vi "Calculate schedules time.vi"(8 "error in (no error)":errorcluster) -> (0 "error out":errorcluster)   [LabVIEW 2020]
uses:
  <vilib>/Utility/miscctls.llb/LVDateTimeRec.ctl
  Global variable.vi
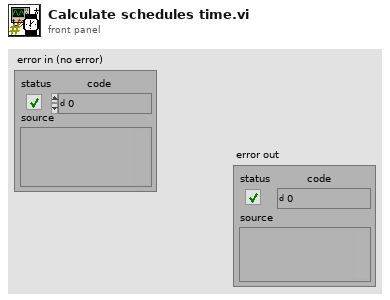
[diagram p1: front panel]
types:
  T1 = typedef "LVDateTimeRec.ctl" = cluster{"fractional second":dbl, "second":i32, "minute":i32, "hour":i32, "day of month":i32, "month":i32, "year":i32, "day of week":i32, "day of year":i32, "DST":i32}
  T2 = typedef "Schedule.ctl" = cluster{"Start time":timestamp, "Repeat":T3, "Action":T4}
  T3 = typedef "Repeat.ctl" = enum16{"None", "Every hour", "Every day", "Every week", "Every month"}
  T4 = typedef "Action.ctl" = u16
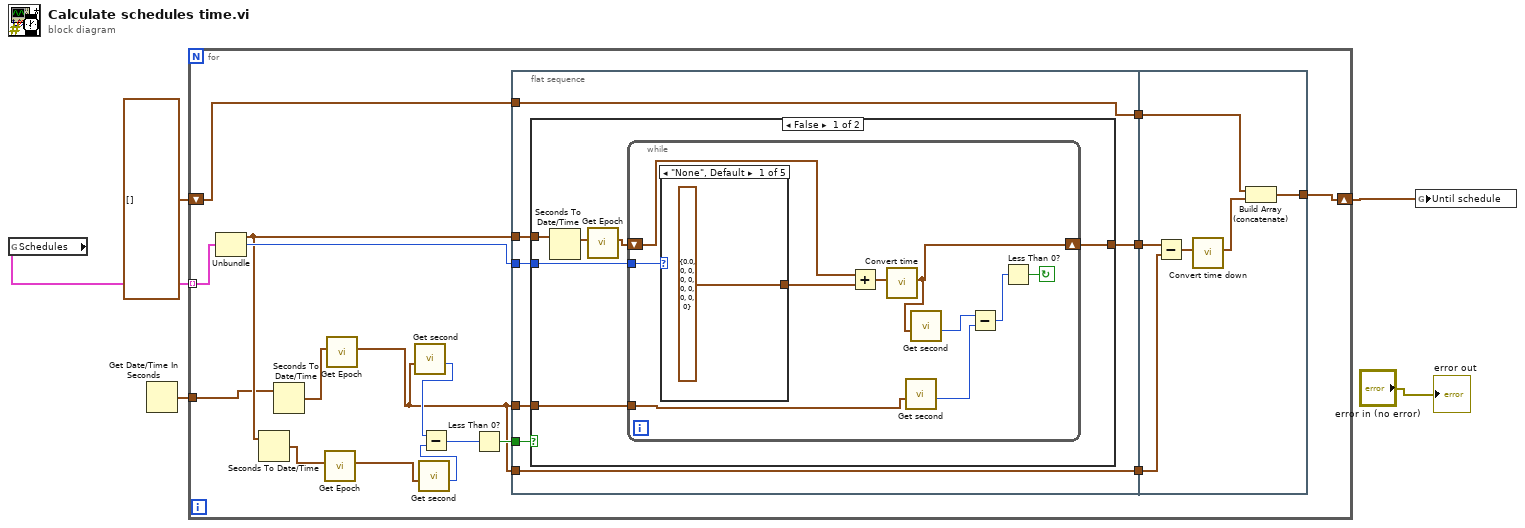
[diagram p0: block diagram]
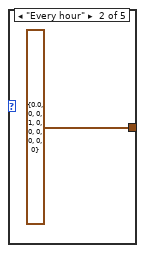
[diagram p2: hidden frame]
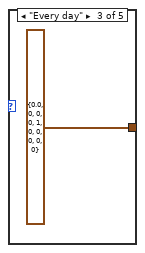
[diagram p3: hidden frame]
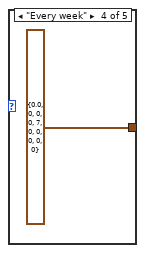
[diagram p4: hidden frame]
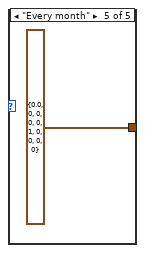
[diagram p5: hidden frame]
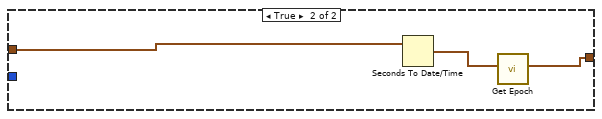
[diagram p6: hidden frame]
diagram:
  n1 = global read "Global variable.vi" "Schedules"() -> (w4:T2[])
  n2 = Get Date/Time In Seconds() -> (seconds since 1Jan1904=w5:timestamp)
  n3 = for {
    tunnel: w4 -> [w22] mode=indexing
    tunnel: w5 -> [w16]
    shift-right: [w15] -> w3
    shift-left: T1[] [] -> [w14]
    n4 = Unbundle(w22) -> ("Start time"=w18:timestamp, "Repeat"=w20:T3)  [unwired: 1 out]
    n5 = Seconds To Date/Time(time stamp (now)=w18) -> (date time rec=w7:T1)  [unwired: 1 in]
    n6 = Seconds To Date/Time(time stamp (now)=w16) -> (date time rec=w8:T1)  [unwired: 1 in]
    n7 = call "Get Epoch.vi"("date time rec 2"=w7) -> ("from epoch"=w6:T1)  [unwired: 9 in, 1 out]
    n8 = call "Get Epoch.vi"("date time rec 2"=w8) -> ("from epoch"=w9:T1)  [unwired: 9 in, 1 out]
    n9 = call "Get second.vi"("date time rec"=w9) -> ("output variable"=w11:i32)  [unwired: 10 in]
    n10 = call "Get second.vi"("date time rec"=w6) -> ("output variable"=w10:i32)  [unwired: 10 in]
    n11 = Subtract(x=w11, y=w10) -> (x-y=w12:i32)
    n12 = Less Than 0?(x=w12) -> (x < 0?=w21:bool)
    n13 = flat-sequence {
      tunnel: w21 -> [w29]
      tunnel: w9 -> [w28]
      tunnel: w18 -> [w27]
      tunnel: w20 -> [w26]
      tunnel: [w25] -> w19
      tunnel: [w24] -> w17
      tunnel: w9 -> [w24]
      tunnel: w14 -> [w23]
      tunnel: [w23] -> w13
      tunnel: w19 -> [w59]
      tunnel: w17 -> [w58]
      tunnel: [w55] -> w15
      tunnel: w13 -> [w54]
      frame #0 {
        n14 = case shown="False" w29 {
          tunnel: w28 -> [w35 _]
          tunnel: w27 -> [w33 w53]
          tunnel: w26 -> [w34 _]
          tunnel: [w32 w52] -> w25
          frame False {
            n15 = Seconds To Date/Time(time stamp (now)=w33) -> (date time rec=w30:T1)  [unwired: 1 in]
            n16 = call "Get Epoch.vi"("date time rec 2"=w30) -> ("from epoch"=w31:T1)  [unwired: 9 in, 1 out]
            n17 = while {
              tunnel: w35 -> [w37]
              shift-right: [w36] -> w32
              shift-left: w31 -> [w42]
              tunnel: w34 -> [w45]
              stop <- w44 continue-if-true
              n18 = case shown="\"None\", Default" w45 {
                tunnel: [T1 {"fractional second"=0.0, "second"=0, "minute"=0, "hour"=0, "day of month"=0, "month"=0, "year"=0, "day of week"=0, "day of year"=0, "DST"=0} ("y") T1 {"fractional second"=0.0, "second"=0, "minute"=0, "hour"=1, "day of month"=0, "month"=0, "year"=0, "day of week"=0, "day of year"=0, "DST"=0} ("y") T1 {"fractional second"=0.0, "second"=0, "minute"=0, "hour"=0, "day of month"=1, "month"=0, "year"=0, "day of week"=0, "day of year"=0, "DST"=0} ("y") T1 {"fractional second"=0.0, "second"=0, "minute"=0, "hour"=0, "day of month"=7, "month"=0, "year"=0, "day of week"=0, "day of year"=0, "DST"=0} ("y") T1 {"fractional second"=0.0, "second"=0, "minute"=0, "hour"=0, "day of month"=0, "month"=1, "year"=0, "day of week"=0, "day of year"=0, "DST"=0} ("y")] -> w43
                frame "None", Default {
                }
                frame "Every hour" {
                }
                frame "Every day" {
                }
                frame "Every week" {
                }
                frame "Every month" {
                }
              }
              n19 = Add(x=w42, y=w43) -> (x+y=w41:T1)
              n20 = call "Convert time.vi"("date time rec"=w41) -> ("date time rec 2"=w36:T1)  [unwired: 10 in]
              n21 = call "Get second.vi"("date time rec"=w37) -> ("output variable"=w39:i32)  [unwired: 10 in]
              n22 = call "Get second.vi"("date time rec"=w36) -> ("output variable"=w40:i32)  [unwired: 10 in]
              n23 = Subtract(x=w40, y=w39) -> (x-y=w38:i32)
              n24 = Less Than 0?(x=w38) -> (x < 0?=w44:bool)
            }
          }
          frame True {
            n25 = Seconds To Date/Time(time stamp (now)=w53) -> (date time rec=w51:T1)  [unwired: 1 in]
            n26 = call "Get Epoch.vi"("date time rec 2"=w51) -> ("from epoch"=w52:T1)  [unwired: 9 in, 1 out]
          }
        }
      }
      frame #1 {
        n27 = Subtract(x=w59, y=w58) -> (x-y=w57:T1)
        n28 = call "Convert time down.vi"("date time rec"=w57) -> ("date time rec 2"=w56:T1)  [unwired: 10 in]
        n29 = Build Array (concatenate)(w54, w56) -> (w55:T1[])
      }
    }
  }
  n30 = global write "Global variable.vi" "Until schedule"(w3) -> ()
  "error out" <- "error in (no error)"
